vi "loose classification compare.vi"(10 "class 2":T1, 11 "class 1":T1) -> (3 "match?":bool)   [LabVIEW 2013, in "engine configuration.lvclass"]
uses:
  engine configuration.lvclass
  <vilib>/NI/Tag Bus Module Framework/channel/channel classification.ctl
  <vilib>/NI/Tag Bus Module Framework/channel/TBM channel.lvclass
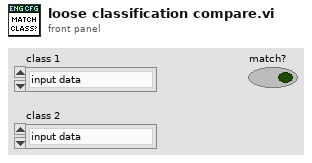
[diagram p1: front panel]
types:
  T1 = typedef "TBM channel.lvclass/channel classification.ctl" = enum16{"input data", "output data", "processing parameter", "processing result"}
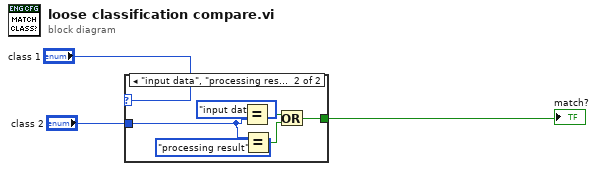
[diagram p0: block diagram]
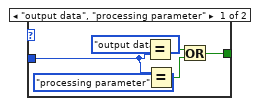
[diagram p2: hidden frame]
diagram:
  n1 = case shown="\"input data\", \"processing result\"" "class 1" {
    tunnel: "class 2" -> [w6 w12]
    tunnel: [w7 w13] -> w3
    frame "output data", "processing parameter" {
      n2 = Equal?(x=channel_classification."output data", y=w6) -> (x = y?=w9:bool)
      n3 = Equal?(x=w6, y=channel_classification."processing parameter") -> (x = y?=w8:bool)
      n4 = Or(x=w9, y=w8) -> (x .or. y?=w7:bool)
    }
    frame "input data", "processing result" {
      n5 = Equal?(x=channel_classification."input data", y=w12) -> (x = y?=w15:bool)
      n6 = Equal?(x=w12, y=channel_classification."processing result") -> (x = y?=w14:bool)
      n7 = Or(x=w15, y=w14) -> (x .or. y?=w13:bool)
    }
  }
  "match?" <- w3
